vi "8.6.vi"() -> ()   [LabVIEW 8.6]
panel:
  out "appended array":dbl[](array[numeric])
  in  "Numeric":dbl
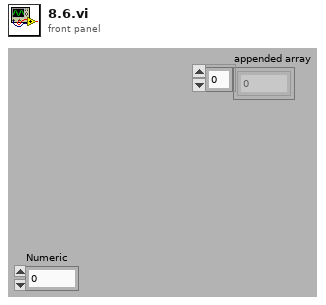
[diagram p1: front panel]
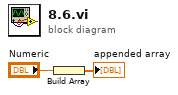
[diagram p0: block diagram]
diagram:
  n1 = Build Array("Numeric") -> (→"appended array":dbl[])
